vi "Ripple.vi"() -> ()   [LabVIEW 2020]
uses:
  pmbus_ltm4676a/controls/ltm4676a_config.ctl
  controls/psrr_nightwing_config.ctl
  controls/psrr_heatwave_config.ctl
  controls/psrr_scope_config.ctl
  <instrlib>/niDCPower/nidcpower.llb/niDCPower Source Mode.ctl
  <instrlib>/niDCPower/nidcpower.llb/niDCPower Output Function.ctl
  <instrlib>/niDCPower/nidcpower.llb/niDCPower Sense.ctl
  <instrlib>/niDCPower/nidcpower.llb/niDCPower Wait For Event - Event.ctl
  <instrlib>/niScope/Controls/niScope vertical coupling.ctl
  <instrlib>/niScope/Controls/niScope trigger slope.ctl
  <instrlib>/niScope/Controls/niScope trigger coupling.ctl
  <instrlib>/niScope/Controls/niScope trigger source.ctl
  <vilib>/Analysis/baseanly.llb/Mean (DBL).vi
  <instrlib>/niScope/Utility/niScope Get Channel Name From String.vi
  <instrlib>/niScope/Configure/Trigger/niScope Configure Trigger Edge.vi
  <vilib>/Analysis/NI_AALBase.lvlib
panel:
  in  "App control":enum32{"Main", "Debug", "Ref"}(tab)
  out "Output Voltage (V) vs. Time (s)":waveform(dbl)[](graph)
  in  "Config control":T1(tab)
  in  "Source config":T2={"Source device name"="PXIe-4139-source", "Source device channel"="0", "Source device voltage (V)"=10.0, "Source current limit (A)"=0.25, "Channel setup time (s)"=0.5} {"Channel setup time (s)" format="%_4p"}
  in  "Load config":T3={"Load device name"="PXIe-4141-load", "Load device channel"="3", "Load device current (A)"=0.075, "Load voltage limit (V)"=6.0, "Channel setup time (s)"=0.5} {"Channel setup time (s)" format="%_4p"}
  in  "Scope config":T4={"Resource name"="Scope", "Scope channel(s)"="0", "Probe Attenuation"=1.0, "Samples per cycle"=10000, "Cycles to acquire"=8} {"Cycles to acquire" min=1 step=1; "Probe Attenuation" format="%.1f"; "Samples per cycle" step=1000000}
  in  "LTM4676A Runtime Config":T5={"SDC config path"=path "C:/Users/Administrator/Documents/qkocian-sandbox/demos/argus-buck-demo/instrumentstudio/sdc/pmbus_ltm4676a.sdconfig", "Output setpoint (V)"=3.3, "Voltage margin (%)"=5.0, "Voltage warn limit (%)"=7.5, "Voltage fault limit (%)"=10.0, "Switching frequency (kHz)"=650} {"Switching frequency (kHz)" items=["250"=62440, "350"=64188, "425"=64338, "500"=64488, "575"=575, "650"=650, "750"=750, "1000"=1000]; "Voltage fault limit (%)" min=0.0 max=100.0 step=1.0 format="%.1g"; "Voltage warn limit (%)" min=0.0 max=100.0 step=1.0 format="%.1g"; "Voltage margin (%)" min=0.0 max=100.0 step=1.0 format="%.1g"; "Output setpoint (V)" min=0.5 max=5.5 step=0.1}
  out "Ripple Voltage (RMS)":dbl[](array[numeric]) format="%.2p"
  out "Ripple Voltage (Peak to Peak)":dbl[](array[numeric]) format="%.2p"
  out "mean":dbl=0.006085820496082306 format="%0.2f"
  out "success?":bool
  in  "Use PMBus?":bool
  out "Actual sample rate":dbl=60000000.0 format="%#.2p"
  out "Actual record length":i32=9600
  out "Actual sample rate":dbl=60000000.0 caption="Requested sample rate" format="%#.2p"
  out "Requested record length":i32=9600
  out "Supply voltage":dbl[](array[numeric])=[9.99999878799602]
  out "Supply current":dbl[](array[numeric])=[0.22298588317976026]
  out "Load voltage":dbl[](array[numeric])=[-3.302483203205584]
  out "Load current":dbl[](array[numeric])=[0.07499996347061717]
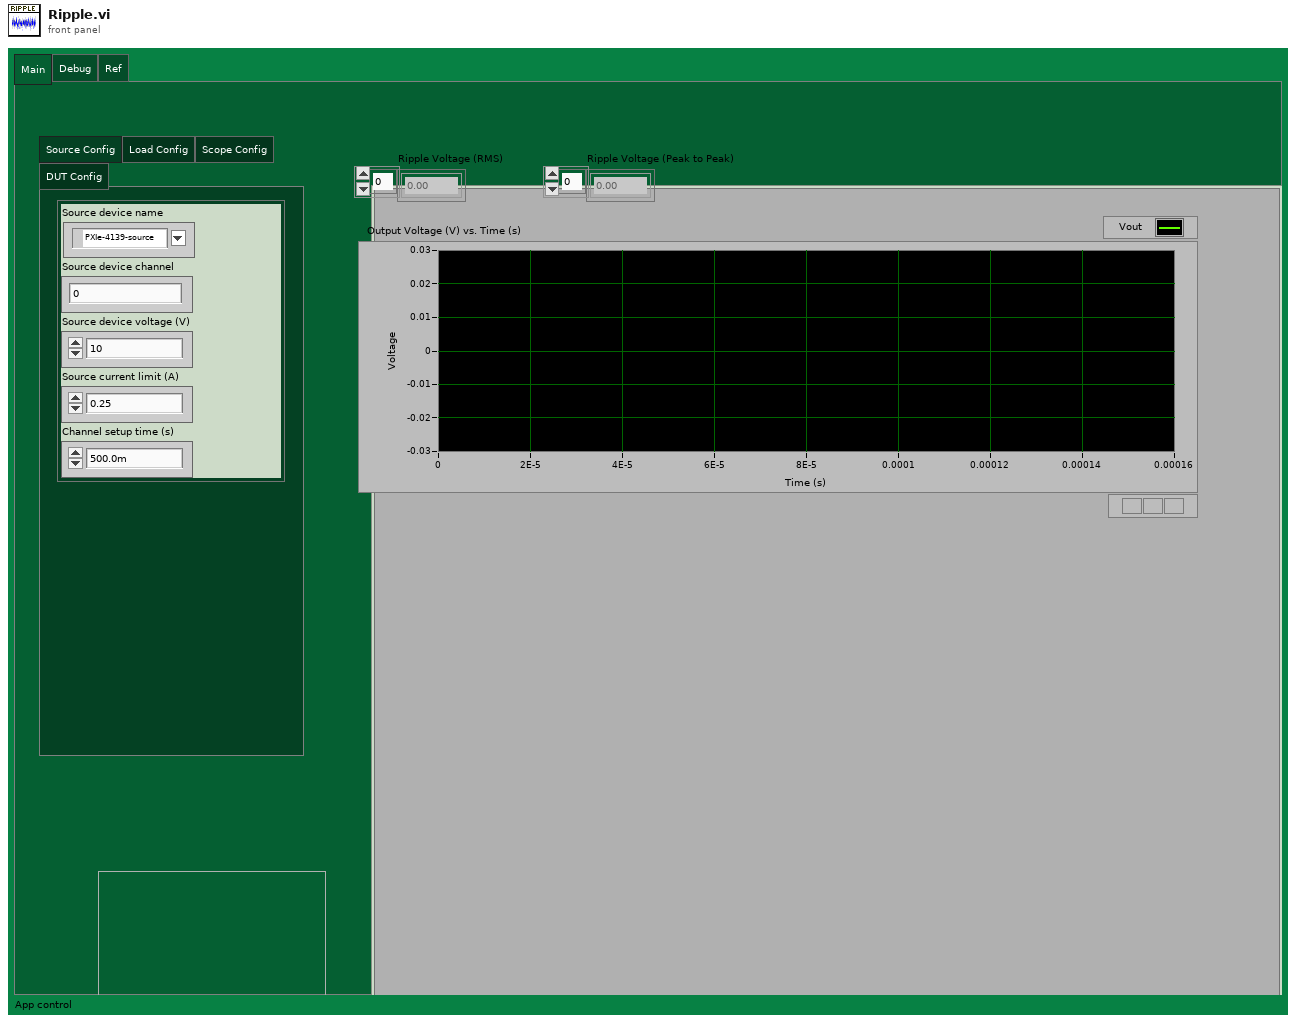
[diagram p1: front panel]
types:
  T1 = enum32{"Source Config", "Load Config", "Scope Config", "DUT Config"}
  T2 = typedef "psrr_nightwing_config.ctl" = cluster{"Source device name":refnum<k15>, "Source device channel":string, "Source device voltage (V)":dbl, "Source current limit (A)":dbl, "Channel setup time (s)":dbl}
  T3 = typedef "psrr_heatwave_config.ctl" = cluster{"Load device name":refnum<k15>, "Load device channel":string, "Load device current (A)":dbl, "Load voltage limit (V)":dbl, "Channel setup time (s)":dbl}
  T4 = typedef "psrr_scope_config.ctl" = cluster{"Resource name":refnum<k15>, "Scope channel(s)":string, "Probe Attenuation":dbl, "Samples per cycle":u32, "Cycles to acquire":u16}
  T5 = typedef "ltm4676a_config.ctl" = cluster{"SDC config path":path, "Output setpoint (V)":dbl, "Voltage margin (%)":dbl, "Voltage warn limit (%)":dbl, "Voltage fault limit (%)":dbl, "Switching frequency (kHz)":u16}
  T6 = typedef "niDCPower Wait For Event - Event.ctl" = i32
  T7 = typedef "niDCPower Sense.ctl" = i32
  T8 = typedef "niDCPower Output Function.ctl" = i32
  T9 = typedef "niDCPower Source Mode.ctl" = i32
  T10 = typedef "niScope trigger source.ctl" = string
  T11 = typedef "niScope trigger coupling.ctl" = u16
  T12 = typedef "niScope trigger slope.ctl" = i32
  T13 = typedef "niScope vertical coupling.ctl" = i32
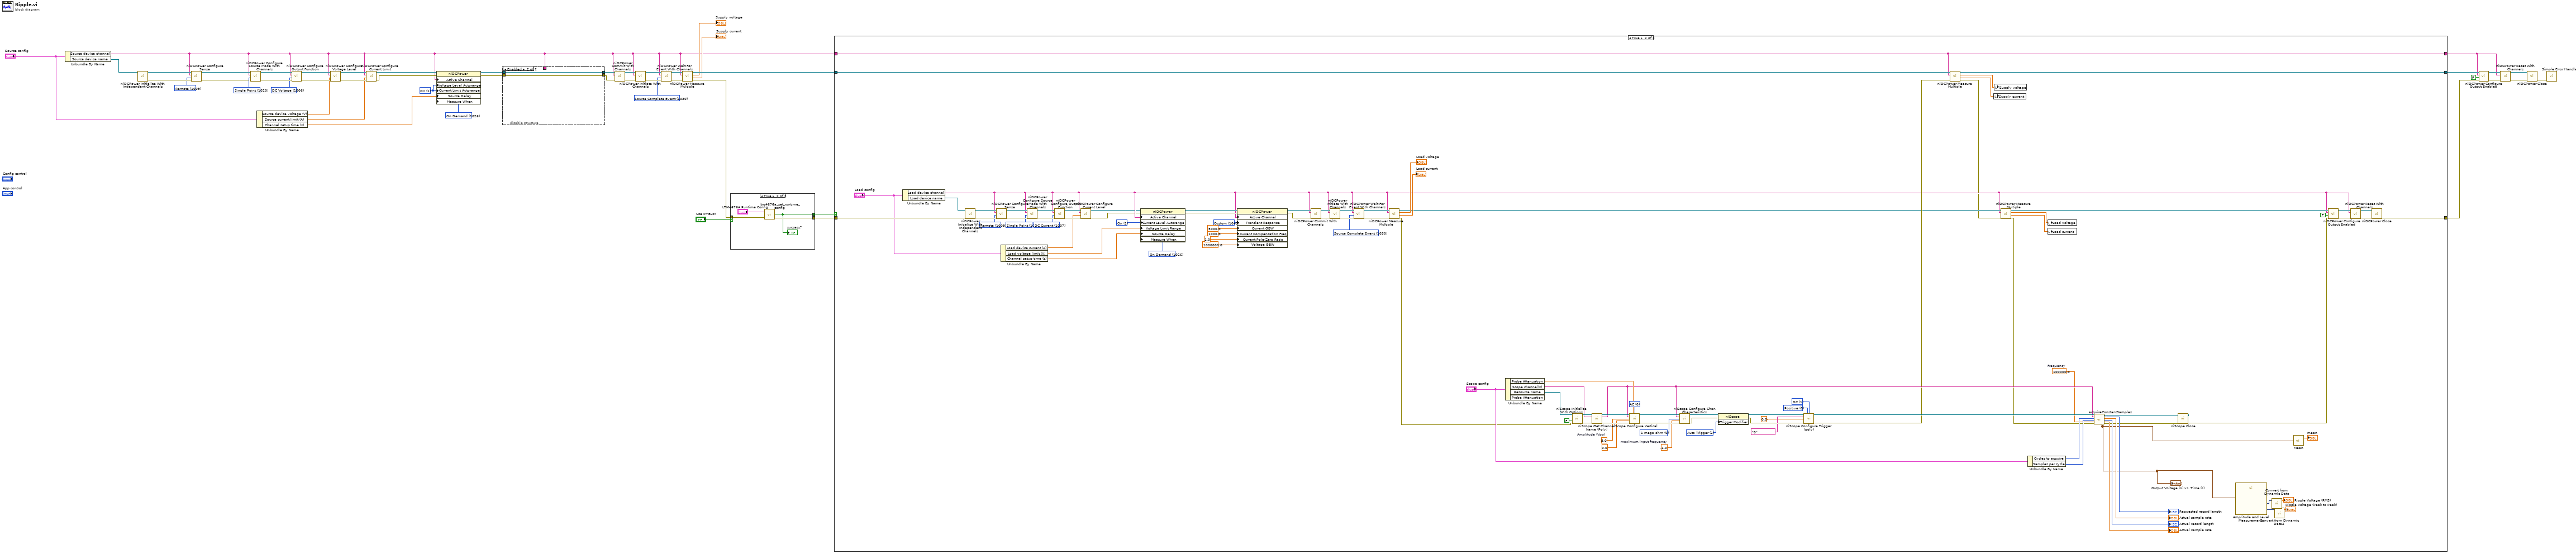
[diagram p0: block diagram]
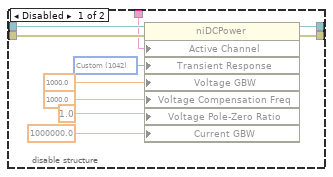
[diagram p2: hidden frame]
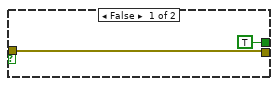
[diagram p3: hidden frame]
diagram:
  w8 = T6 1030 items=["Source Complete Event"=1030, "Measure Complete Event"=1031, "Sequence Iteration Complete Event"=1032, "Sequence Engine Done Event"=1033, "Pulse Complete Event"=1051, "Ready For Pulse Trigger Event"=1052] ("event")
  w33 = T7 1009 items=["Local"=1008, "Remote"=1009] ("sense")
  w36 = 1026 items=["Automatically after Source Complete"=1025, "On Demand"=1026, "On Measure Trigger"=1027] ("Measurement:Advanced:Measure When")
  w45 = 1 items=["Off", "On"] ("Source:DC Voltage:Current Limit Autorange")
  w47 = T8 1006 items=["DC Voltage"=1006, "DC Current"=1007, "Pulse Voltage"=1049, "Pulse Current"=1050] ("output function")
  w50 = T9 1020 items=["Single Point"=1020, "Sequence"=1021] ("source mode")
  n1 = Unbundle By Name("Source config") -> ("Source device channel"=w1:string, "Source device name"=w26:refnum<k15>)
  n2 = call <instrlib>:"niDCPower Initialize With Independent Channels.vi"("resource name"=w26) -> ("error out"=w34:errorcluster, "instrument handle out"=w35:refnum<k15>)  [unwired: 9 in]
  n3 = call <instrlib>:"niDCPower Configure Sense.vi"("error in (no error)"=w34, "sense"=w33, "channel name"=w1, "instrument handle"=w35) -> ("error out"=w25:errorcluster, "instrument handle out"=w24:refnum<k15>)  [unwired: 6 in]
  n4 = call <instrlib>:"niDCPower Configure Source Mode With Channels.vi"("error in (no error)"=w25, "source mode"=w50, "channel name"=w1, "instrument handle"=w24) -> ("error out"=w49:errorcluster, "instrument handle out"=w48:refnum<k15>)  [unwired: 6 in]
  n5 = Unbundle By Name("Source config") -> ("Source device voltage (V)"=w13:dbl, "Source current limit (A)"=w14:dbl, "Channel setup time (s)"=w12:dbl)
  n6 = call <instrlib>:"niDCPower Configure Output Function.vi"("error in (no error)"=w49, "output function"=w47, "channel name"=w1, "instrument handle"=w48) -> ("error out"=w40:errorcluster, "instrument handle out"=w39:refnum<k15>)  [unwired: 6 in]
  n7 = call <instrlib>:"niDCPower Configure Voltage Level.vi"("error in (no error)"=w40, "voltage level"=w13, "channel name"=w1, "instrument handle"=w39) -> ("error out"=w37:errorcluster, "instrument handle out"=w38:refnum<k15>)  [unwired: 6 in]
  n8 = call <instrlib>:"niDCPower Configure Current Limit.vi"("error in (no error)"=w37, "current limit"=w14, "channel name"=w1, "instrument handle"=w38) -> ("error out"=w46:errorcluster, "instrument handle out"=w44:refnum<k15>)  [unwired: 6 in]
  n9 = property class="niDCPower"(reference=w44, error in=w46, "Active Channel"=w1, "Voltage Level Autorange"=w45, "Current Limit Autorange"=w45, "Source Delay"=w12, "Measure When"=w36) -> (reference out=w30:refnum<k15>, error out=w29:errorcluster)
  n10 = disable-structure shown="Enabled" {
    disable-tunnel: w30 -> [w60 w62]
    disable-tunnel: w29 -> [w59 w61]
    disable-tunnel: [w58 w62] -> w28
    disable-tunnel: [w57 w61] -> w27
    disable-tunnel: w1 -> [w56 _]
    frame Disabled {
      w55 = 1042 items=["Slow"=1041, "Normal"=1038, "Fast"=1039, "Custom"=1042] ("Source:Transient Response")
      n11 = property class="niDCPower"(reference=w60, error in=w59, "Active Channel"=w56, "Transient Response"=w55, "Voltage GBW"=1000.0 ("Source:Custom Transient Response:Voltage:Gain Bandwidth"), "Voltage Compensation Freq"=1000.0 ("Source:Custom Transient Response:Voltage:Compensation Frequency"), "Voltage Pole-Zero Ratio"=1.0 ("Source:Custom Transient Response:Voltage:Pole-Zero Ratio"), "Current GBW"=1000000.0 ("Source:Custom Transient Response:Current:Gain Bandwidth")) -> (reference out=w58:refnum<k15>, error out=w57:errorcluster)
    }
    frame Enabled {
    }
  }
  n12 = call <instrlib>:"niDCPower Commit With Channels.vi"("error in (no error)"=w27, "channel name"=w1, "instrument handle"=w28) -> ("error out"=w31:errorcluster, "instrument handle out"=w32:refnum<k15>)  [unwired: 7 in]
  n13 = call <instrlib>:"niDCPower Initiate With Channels.vi"("error in (no error)"=w31, "channel name"=w1, "instrument handle"=w32) -> ("error out"=w9:errorcluster, "instrument handle out"=w10:refnum<k15>)  [unwired: 7 in]
  n14 = call <instrlib>:"niDCPower Wait For Event With Channels.vi"("error in (no error)"=w9, "event"=w8, "channel name"=w1, "instrument handle"=w10) -> ("error out"=w7:errorcluster, "instrument handle out"=w6:refnum<k15>)  [unwired: 6 in]
  n15 = call <instrlib>:"niDCPower Measure Multiple.vi"("error in (no error)"=w7, "channel name"=w1, "instrument handle"=w6) -> ("error out"=w5:errorcluster, "current measurements"=→"Supply current":dbl[], "voltage measurements"=→"Supply voltage":dbl[], "instrument handle out"=w4:refnum<k15>)  [unwired: 5 in]
  n16 = case shown="True" "Use PMBus?" {
    tunnel: [w64 w68] -> w23
    tunnel: w5 -> [w64 w67]
    tunnel: [TRUE ("success?") w66] -> w19
    frame False {
    }
    frame True {
      n17 = call "ltm4676a_set_runtime_config.vi"("LTM4676A Runtime Config"="LTM4676A Runtime Config", "error in (no error)"=w67) -> ("success?"=w66:bool, "error out"=w68:errorcluster)  [unwired: 1 out]
      "success?" <- w66
    }
  }
  n18 = case shown="True" w19 {
    tunnel: w23 -> [w69 w161]
    tunnel: [w69 w127] -> w11
    tunnel: w4 -> [w71 w107]
    tunnel: [w71 w105] -> w18
    tunnel: w1 -> [w70 w106]
    tunnel: [w70 w106] -> w17
    frame False {
    }
    frame True {
      w80 = -1.0  # maximum input frequency
      w87 = 100000.0  # Frequency
      w98 = 5.0  # Amplitude (Vpp)
      w109 = T8 1007 items=["DC Voltage"=1006, "DC Current"=1007, "Pulse Voltage"=1049, "Pulse Current"=1050] ("output function")
      w110 = T9 1020 items=["Single Point"=1020, "Sequence"=1021] ("source mode")
      w112 = 1026 items=["Automatically after Source Complete"=1025, "On Demand"=1026, "On Measure Trigger"=1027] ("Measurement:Advanced:Measure When")
      w139 = 2 items=["None"=1, "Auto Trigger"=2] ("Triggering:Trigger Modifier")
      w85 = T11 1 items=["AC"=0, "DC"=1, "HF Reject"=3, "LF Reject"=4, "AC Plus HF Reject"=1001] ("trigger coupling")
      w86 = T12 0 items=["Positive", "Negative"] ("trigger slope")
      w82 = T13 0 items=["AC", "DC", "Ground"] ("vertical coupling")
      w148 = u32 0 items=["1 mega ohm"=0, "50 ohms"=2] ("input impedance")
      w113 = 1 items=["Off", "On"] ("Source:DC Current:Current Level Autorange")
      w164 = 1042 items=["Slow"=1041, "Normal"=1038, "Fast"=1039, "Custom"=1042] ("Source:Transient Response")
      w167 = T6 1030 items=["Source Complete Event"=1030, "Measure Complete Event"=1031, "Sequence Iteration Complete Event"=1032, "Sequence Engine Done Event"=1033, "Pulse Complete Event"=1051, "Ready For Pulse Trigger Event"=1052] ("event")
      w170 = T7 1009 items=["Local"=1008, "Remote"=1009] ("sense")
      n19 = Unbundle By Name("Load config") -> ("Load device channel"=w103:string, "Load device name"=w162:refnum<k15>)
      n20 = call <instrlib>:"niDCPower Initialize With Independent Channels.vi"("error in (no error)"=w161, "resource name"=w162) -> ("error out"=w172:errorcluster, "instrument handle out"=w171:refnum<k15>)  [unwired: 8 in]
      n21 = call <instrlib>:"niDCPower Configure Sense.vi"("error in (no error)"=w172, "sense"=w170, "channel name"=w103, "instrument handle"=w171) -> ("error out"=w116:errorcluster, "instrument handle out"=w119:refnum<k15>)  [unwired: 6 in]
      n22 = Unbundle By Name("Load config") -> ("Load device current (A)"=w111:dbl, "Load voltage limit (V)"=w100:dbl, "Channel setup time (s)"=w155:dbl)
      n23 = call <instrlib>:"niDCPower Configure Source Mode With Channels.vi"("error in (no error)"=w116, "source mode"=w110, "channel name"=w103, "instrument handle"=w119) -> ("error out"=w115:errorcluster, "instrument handle out"=w118:refnum<k15>)  [unwired: 6 in]
      n24 = call <instrlib>:"niDCPower Configure Output Function.vi"("error in (no error)"=w115, "output function"=w109, "channel name"=w103, "instrument handle"=w118) -> ("error out"=w114:errorcluster, "instrument handle out"=w117:refnum<k15>)  [unwired: 6 in]
      n25 = call <instrlib>:"niDCPower Configure Current Level.vi"("error in (no error)"=w114, "current level"=w111, "channel name"=w103, "instrument handle"=w117) -> ("error out"=w101:errorcluster, "instrument handle out"=w102:refnum<k15>)  [unwired: 6 in]
      n26 = property class="niDCPower"(reference=w102, error in=w101, "Active Channel"=w103, "Current Level Autorange"=w113, "Voltage Limit Range"=w100, "Source Delay"=w155, "Measure When"=w112) -> (reference out=w160:refnum<k15>, error out=w159:errorcluster)
      n27 = property class="niDCPower"(reference=w160, error in=w159, "Active Channel"=w103, "Transient Response"=w164, "Current GBW"=5000.0 ("Source:Custom Transient Response:Current:Gain Bandwidth"), "Current Compensation Freq"=1000.0 ("Source:Custom Transient Response:Current:Gain Bandwidth"), "Current Pole-Zero Ratio"=1.0 ("Source:Custom Transient Response:Current:Gain Bandwidth"), "Voltage GBW"=1000000.0 ("Source:Custom Transient Response:Voltage:Gain Bandwidth")) -> (reference out=w125:refnum<k15>, error out=w124:errorcluster)
      n28 = call <instrlib>:"niDCPower Commit With Channels.vi"("error in (no error)"=w124, "channel name"=w103, "instrument handle"=w125) -> ("error out"=w165:errorcluster, "instrument handle out"=w166:refnum<k15>)  [unwired: 7 in]
      n29 = call <instrlib>:"niDCPower Initiate With Channels.vi"("error in (no error)"=w165, "channel name"=w103, "instrument handle"=w166) -> ("error out"=w169:errorcluster, "instrument handle out"=w168:refnum<k15>)  [unwired: 7 in]
      n30 = call <instrlib>:"niDCPower Wait For Event With Channels.vi"("error in (no error)"=w169, "event"=w167, "channel name"=w103, "instrument handle"=w168) -> ("error out"=w122:errorcluster, "instrument handle out"=w123:refnum<k15>)  [unwired: 6 in]
      n31 = call <instrlib>:"niDCPower Measure Multiple.vi"("error in (no error)"=w122, "channel name"=w103, "instrument handle"=w123) -> ("error out"=w99:errorcluster, "current measurements"=→"Load current":dbl[], "voltage measurements"=→"Load voltage":dbl[], "instrument handle out"=w104:refnum<k15>)  [unwired: 5 in]
      n32 = Unbundle By Name("Scope config") -> ("Probe Attenuation"=w138:dbl, "Scope channel(s)"=w144:string, "Resource name"=w145:refnum<k15>)  [unwired: 1 out]
      n33 = call <instrlib>:"niScope Initialize With Options.vi"("resource name"=w145, "reset device"=FALSE, "error in"=w99) -> ("instrument handle"=w154:refnum<k15>, "error out"=w151:errorcluster)  [unwired: 11 in]
      n34 = call-poly <instrlib>:"niScope Get Channel Name (Poly).vi"("instrument handle"=w154, "index"=w144, "error in"=w151) -> ("instrument handle out"=w153:refnum<k15>, "channel name"=w133:string, "error out"=w150:errorcluster)  [unwired: 10 in]
      n35 = call <instrlib>:"niScope Configure Vertical.vi"("instrument handle"=w153, "probe attenuation"=w138, "vertical coupling"=w82, "channels"=w133, "vertical range"=w98, "vertical offset"=0.0, "error in"=w150) -> ("instrument handle out"=w152:refnum<k15>, "error out"=w149:errorcluster)  [unwired: 7 in]
      n36 = call <instrlib>:"niScope Configure Chan Characteristics.vi"("instrument handle"=w152, "channels"=w133, "input impedance"=w148, "maximum input frequency"=w80, "error in"=w149) -> ("instrument handle out"=w143:refnum<k15>, "error out"=w142:errorcluster)  [unwired: 9 in]
      n37 = property on="Property Node" class="niScope"(reference=w143, error in=w142, "Trigger Modifier"=w139) -> (reference out=w141:refnum<k15>, error out=w140:errorcluster)
      n38 = call-poly <instrlib>:"niScope Configure Trigger (poly).vi"("instrument handle"=w141, "trigger slope"=w86, "trigger coupling"=w85, "trigger source"=T10 "0", "trigger level"=0.0, "error in"=w140) -> ("instrument handle out"=w137:refnum<k15>, "error out"=w108:errorcluster)  [unwired: 8 in]
      n39 = call <instrlib>:"niDCPower Measure Multiple.vi"("error in (no error)"=w108, "channel name"=w106, "instrument handle"=w107) -> ("error out"=w93:errorcluster, "current measurements"=w91:dbl[], "voltage measurements"=w92:dbl[], "instrument handle out"=w105:refnum<k15>)  [unwired: 5 in]
      n40 = local write "Supply current"(w91) -> ()
      n41 = local write "Supply voltage"(w92) -> ()
      n42 = call <instrlib>:"niDCPower Measure Multiple.vi"("error in (no error)"=w93, "channel name"=w103, "instrument handle"=w104) -> ("error out"=w88:errorcluster, "current measurements"=w89:dbl[], "voltage measurements"=w90:dbl[])  [unwired: 5 in, 1 out]
      n43 = Unbundle By Name("Scope config") -> ("Cycles to acquire"=w135:u16, "Samples per cycle"=w134:u32)
      n44 = local write "Load voltage"(w90) -> ()
      n45 = local write "Load current"(w89) -> ()
      n46 = call "acquireConstantSamples.vi"("Instrument handle"=w137, "Channel(s)"=w133, "Cycles to acquire"=w135, "Samples/cycle"=w134, "Frequency"=w87, "error in (no error)"=w88) -> ("Waveform(s)"=w74:waveform(dbl)[], "Instrument handle out"=w73:refnum<k15>, "Requested record length"=→"Requested record length":i32, "Reqested sample rate"=→"Actual sample rate":dbl, "Actual record length"=→"Actual record length":i32, "Actual sample rate"=→"Actual sample rate":dbl, "error out"=w72:errorcluster)  [unwired: 7 in]
      "Output Voltage (V) vs. Time (s)" <- w74
      n47 = call <instrlib>:"niScope Close.vi"("instrument handle"=w73, "error in"=w72) -> ("error out"=w79:errorcluster)  [unwired: 13 in]
      n48 = call "Amplitude and Level Measurements"("Signals"=w74) -> ("RMS"=w78:dynamicdata, "Peak to Peak"=w76:dynamicdata)  [unwired: 12 in, 1 out]
      n49 = call "Convert from Dynamic Data"("Dynamic Data Type"=w78) -> ("Array"=→"Ripple Voltage (RMS)":dbl[])  [unwired: 3 in]
      n50 = call "Convert from Dynamic Data2"("Dynamic Data Type"=w76) -> ("Array"=→"Ripple Voltage (Peak to Peak)":dbl[])  [unwired: 3 in]
      n51 = call-poly <vilib>:"Mean.vi"("X"=w74) -> ("mean"=→"mean":dbl)  [unwired: 1 out]
      n52 = call <instrlib>:"niDCPower Configure Output Enabled.vi"("error in (no error)"=w79, "output enabled"=FALSE, "channel name"=w103, "instrument handle"=w104) -> ("error out"=w132:errorcluster, "instrument handle out"=w131:refnum<k15>)  [unwired: 6 in]
      n53 = call <instrlib>:"niDCPower Reset With Channels.vi"("error in (no error)"=w132, "channel name"=w103, "instrument handle"=w131) -> ("error out"=w129:errorcluster, "instrument handle out"=w130:refnum<k15>)  [unwired: 7 in]
      n54 = call <instrlib>:"niDCPower Close.vi"("error in (no error)"=w129, "instrument handle"=w130) -> ("error out"=w127:errorcluster)  [unwired: 9 in]
    }
  }
  n55 = call <instrlib>:"niDCPower Configure Output Enabled.vi"("error in (no error)"=w11, "output enabled"=FALSE, "channel name"=w17, "instrument handle"=w18) -> ("error out"=w20:errorcluster, "instrument handle out"=w21:refnum<k15>)  [unwired: 6 in]
  n56 = call <instrlib>:"niDCPower Reset With Channels.vi"("error in (no error)"=w20, "channel name"=w17, "instrument handle"=w21) -> ("error out"=w42:errorcluster, "instrument handle out"=w43:refnum<k15>)  [unwired: 7 in]
  n57 = call <instrlib>:"niDCPower Close.vi"("error in (no error)"=w42, "instrument handle"=w43) -> ("error out"=w41:errorcluster)  [unwired: 9 in]
  n58 = call <vilib>:"Simple Error Handler.vi"("error in (no error)"=w41) -> ()  [unwired: 4 in, 5 out]
